vi "Video Toolset Stop.vi"   [LabVIEW 2010]
types:
  T1 = enum32{"Bad", "Idle", "Run top level", "Running"}
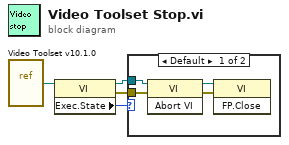
[diagram p0: block diagram]
diagram:
  n1 = vi-ref "Video Toolset v10.1.0.vi"() -> (w4:refnum<vi>)
  n2 = property class="VI"(reference=w4) -> (reference out=w3:refnum<vi>, error out=w1:errorcluster, "Exec.State"=w2:T1)  [unwired: 1 in]
  n3 = case shown="Default" w2 {
    tunnel: w3 -> [w8 _]
    tunnel: w1 -> [w5 _]
    frame Default {
      n4 = invoke on="Invoke Node" class="VI" method="Abort VI"(reference=w8, error in=w5) -> (reference out=w7:refnum<vi>, error out=w6:errorcluster)  [unwired: 1 in, 1 out]
      n5 = invoke on="Invoke Node" class="VI" method="FP.Close"(reference=w7, error in=w6) -> ()  [unwired: 1 in, 3 out]
    }
    frame "Bad", "Idle" {
    }
  }
